vi "Ejercicio_7_Histrograma_Arduino.vi"() -> ()   [LabVIEW 2020]
uses:
  <vilib>/Instr/_visa.llb/VISA Configure Serial Port (Instr).vi
  <vilib>/ptbypt/NI_PtbyPt.lvlib
panel:
  in  "sample length":i32=100
  out "Histogram Graph":T1(graph)
  in  "stop":bool
  out "read buffer":string
  in  "VISA resource name":refnum<visa-resource-name>
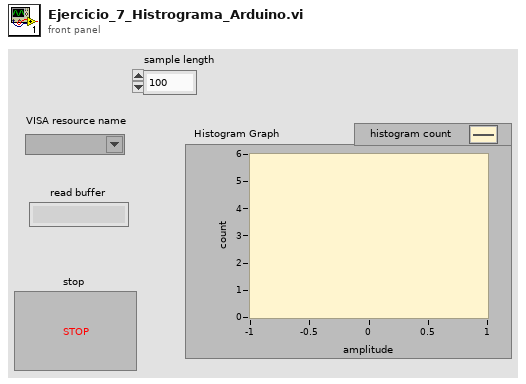
[diagram p1: front panel]
types:
  T1 = cluster{"X Values":dbl[], "Histogram: h(x)":i32[]}
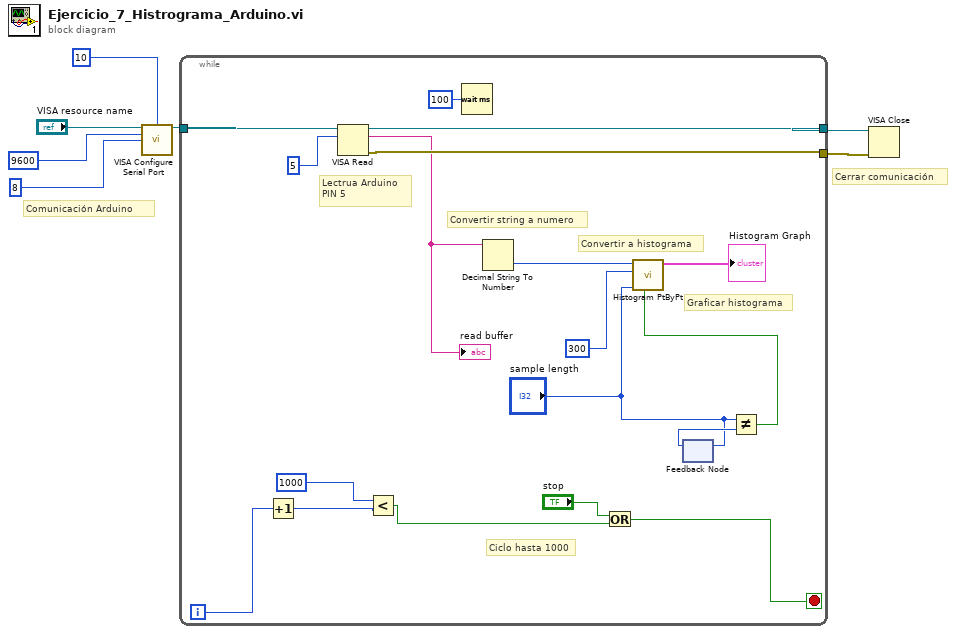
[diagram p0: block diagram]
diagram:
  # "Cerrar comunicación"
  # "Comunicación Arduino"
  n1 = call-poly "VISA Configure Serial Port"("VISA resource name"="VISA resource name", "termination char\n(0xA = '\\n' = LF)"=u8 10 ("termination char\n(0xA = '\\n' = LF)"), "baud rate (9600)"=u32 9600, "data bits (8)"=u16 8) -> ("VISA resource name out"=w4:refnum<visa-resource-name>)  [unwired: 10 in, 1 out]
  n2 = while {
    tunnel: w4 -> [w25]
    tunnel: [w24] -> w3
    tunnel: [w23] -> w2
    i -> [w14]
    stop <- w16 stop-if-true
    # "Graficar histograma"
    # "Convertir a histograma"
    # "Convertir string a numero"
    # "Ciclo hasta 1000"
    # "Lectrua Arduino \nPIN 5"
    n3 = Increment(x=w14) -> (x+1=w13:i32)
    n4 = VISA Read(VISA resource name=w25, byte count=u32 5) -> (VISA resource name out=w24:refnum<visa-resource-name>, read buffer=w9:string, error out=w23:errorcluster)  [unwired: 1 in, 1 out]
    "read buffer" <- w9
    n5 = Less?(x=1000, y=w13) -> (x < y?=w15:bool)
    n6 = Wait (ms)(milliseconds to wait=u32 100) -> ()  [unwired: 1 out]
    n7 = Decimal String To Number(string=w9) -> (number=w8:i32)  [unwired: 2 in, 1 out]
    n8 = Or(x="stop", y=w15) -> (x .or. y?=w16:bool)
    n9 = feedback-in #1("sample length") -> ()
    n10 = feedback #1() -> (w12:i32)  [unwired: 1 in]
    n11 = Not Equal?(x="sample length", y=w12) -> (x != y?=w10:bool)
    n12 = call <vilib>:"Histogram PtByPt.vi"("initialize"=w10, "sample length"="sample length", "intervals"=300, "x"=w8) -> ("Histogram Graph"=→"Histogram Graph":T1)  [unwired: 4 in, 3 out]
  }
  n13 = VISA Close(VISA resource name=w3, error in (no error)=w2) -> ()  [unwired: 1 out]
